vi "ULx Create Channel (CI-Frequency).vi"(0 "task in":refnum<k24>, 5 "counters":refnum<k21>, 9 "units":i32(ring) items=["Hz", "Ticks"], 11 "error in":errorcluster, 13 "starting edge":i32(ring) items=["Rising", "Falling"], 14 "measurement time":dbl=0.01 format="%.3f") -> (4 "task out":refnum<k24>, 15 "error out":errorcluster)   [LabVIEW 2020]
doc: "Creates a channel(s) to measure the frequency of a digital signals."
uses:
  C:/Users/William/Documents/LV 2020 builds/LeaktestDAQ/Source-v33/ULx_LV.dll
  ULx_LV.dll
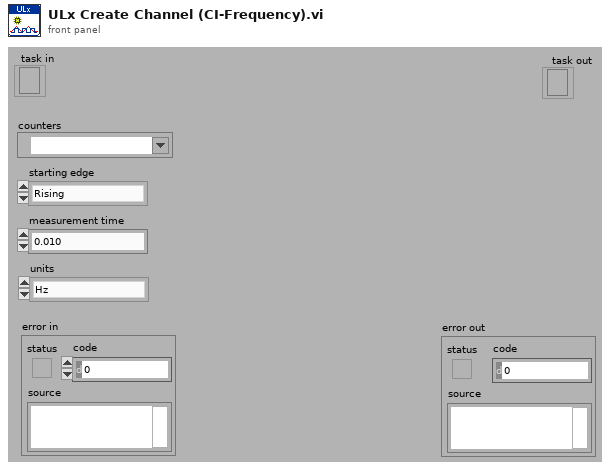
[diagram p1: front panel]
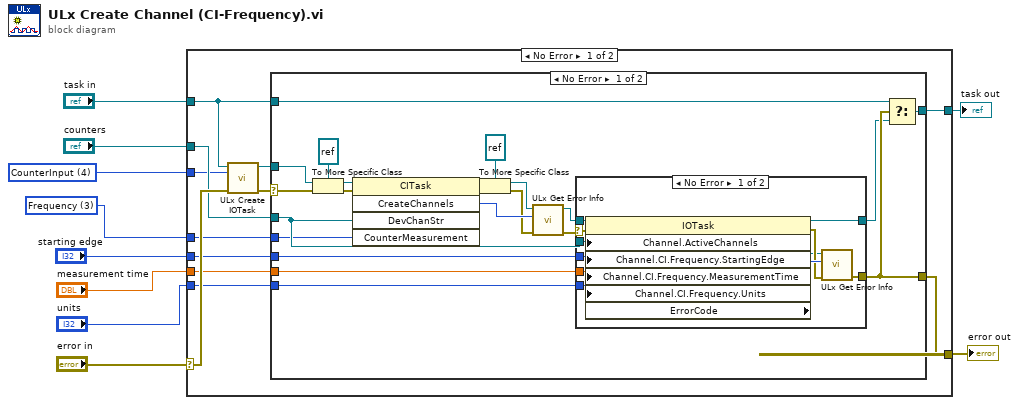
[diagram p0: block diagram]
diagram:
  w1 = 3 items=["CountEdges"=1, "Encoder"=2, "Frequency"=3, "Period"=4] ("CounterMeasurement")
  w6 = 4 items=["AnalogInput", "AnalogOutput", "DigitalInput", "DigitalOutput", "CounterInput", "CounterOutput", "CompositeInput", "CompositeOutput", "TemperatureInput"] ("taskType")
  n1 = case shown="No Error" "error in" {
    selector: "error in" -> [w22 w59]
    tunnel: "task in" -> [w12 w58]
    tunnel: "counters" -> [w17 _]
    tunnel: [w20 w58] -> w8
    tunnel: [w19 w59] -> w7
    tunnel: w6 -> [w16 _]
    tunnel: "starting edge" -> [w15 _]
    tunnel: "measurement time" -> [w14 _]
    tunnel: "units" -> [w13 _]
    tunnel: w1 -> [w11 _]
    frame No Error {
      n2 = call "ULx Create IOTask.vi"("error in"=w22, "taskType"=w16, "i/o task in"=w12) -> ("error out"=w21:errorcluster, "i/o task out"=w18:refnum<k24>)  [unwired: 7 in]
      n3 = case shown="No Error" w21 {
        selector: w21 -> [w41 w57]
        tunnel: [w26 w57] -> w19
        tunnel: [w27 w56] -> w20
        tunnel: w18 -> [w39 _]
        tunnel: w17 -> [w36 _]
        tunnel: w15 -> [w34 _]
        tunnel: w14 -> [w35 _]
        tunnel: w13 -> [w33 _]
        tunnel: w12 -> [w24 w56]
        tunnel: w11 -> [w23 _]
        frame No Error {
          n4 = To More Specific Class(target class=refnum<k24> refnum, reference=w39, error in=w41) -> (specific class reference=w42:refnum<k24>, error out=w40:errorcluster)
          n5 = invoke class="CITask" method="CreateChannels"(reference=w42, error in=w40, "DevChanStr"=w36, "CounterMeasurement"=w23) -> (reference out=w31:refnum<k24>, error out=w30:errorcluster, "CreateChannels"=w38:i32)  [unwired: 1 in, 2 out]
          n6 = To More Specific Class(target class=refnum<k24> refnum, reference=w31, error in=w30) -> (specific class reference=w28:refnum<k24>, error out=w29:errorcluster)
          n7 = call "ULx Get Error Info.vi"("error in"=w29, "ErrorCode"=w38, "task in"=w28) -> ("error out"=w37:errorcluster)  [unwired: 8 in]
          n8 = case shown="No Error" w37 {
            selector: w37 -> [w53 w55]
            tunnel: w28 -> [w52 w54]
            tunnel: w36 -> [w51 _]
            tunnel: [w48 w55] -> w26
            tunnel: w35 -> [w47 _]
            tunnel: w34 -> [w46 _]
            tunnel: w33 -> [w45 _]
            tunnel: [w44 w54] -> w25
            frame No Error {
              n9 = property class="IOTask"(reference=w52, error in=w53, "Channel.ActiveChannels"=w51, "Channel.CI.Frequency.StartingEdge"=w46, "Channel.CI.Frequency.MeasurementTime"=w47, "Channel.CI.Frequency.Units"=w45) -> (reference out=w44:refnum<k24>, error out=w49:errorcluster, "ErrorCode"=w50:i32)
              n10 = call "ULx Get Error Info.vi"("error in"=w49, "ErrorCode"=w50, "task in"=w44) -> ("error out"=w48:errorcluster)  [unwired: 8 in]
            }
            frame Error {
            }
          }
          n11 = Select(t=w24, s=w26, f=w25) -> (s? t:f=w27:refnum<k24>)
        }
        frame Error {
        }
      }
    }
    frame Error {
    }
  }
  "error out" <- w7
  "task out" <- w8
